vi "Check for change in Image Sizes.vi"(9 "Other optical path [Current ImRef]":T1, 10 "Current Optical Path [New ImRef]":T1, 11 "Current Optical Path [Current ImRef]":T1) -> (2 "Other Optical Path [New ImRef] OUT":T1, 3 "Current Optical Path [New ImRef] OUT":T1)   [LabVIEW 2012]
uses:
  <vilib>/vision/Image Controls.llb/IMAQ Image.ctl
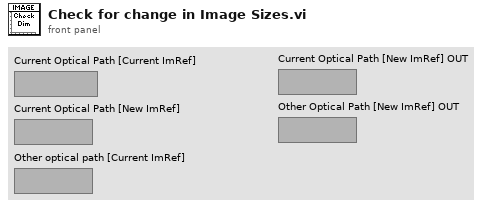
[diagram p1: front panel]
types:
  T1 = typedef "IMAQ Image.ctl" = refnum<image>
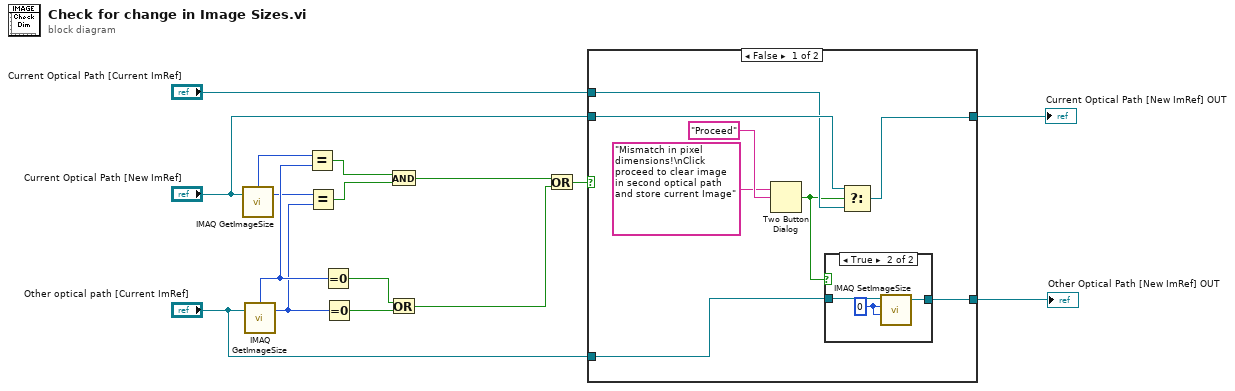
[diagram p0: block diagram]
diagram:
  n1 = call "IMAQ GetImageSize"("Image"="Current Optical Path [New ImRef]") -> ("Y Resolution"=w12:i32, "X Resolution"=w14:i32)  [unwired: 3 in, 1 out]
  n2 = call "IMAQ GetImageSize"("Image"="Other optical path [Current ImRef]") -> ("Y Resolution"=w11:i32, "X Resolution"=w13:i32)  [unwired: 3 in, 1 out]
  n3 = Equal?(x=w14, y=w13) -> (x = y?=w10:bool)
  n4 = Equal?(x=w12, y=w11) -> (x = y?=w9:bool)
  n5 = Equal To 0?(x=w13) -> (x = 0?=w16:bool)
  n6 = Equal To 0?(x=w11) -> (x = 0?=w15:bool)
  n7 = And(x=w10, y=w9) -> (x .and. y?=w8:bool)
  n8 = Or(x=w16, y=w15) -> (x .or. y?=w7:bool)
  n9 = Or(x=w8, y=w7) -> (x .or. y?=w6:bool)
  n10 = case shown="False" w6 {
    tunnel: "Current Optical Path [Current ImRef]" -> [w21 _]
    tunnel: "Current Optical Path [New ImRef]" -> [w22 w29]
    tunnel: "Other optical path [Current ImRef]" -> [w19 w30]
    tunnel: [w18 w30] -> w2
    tunnel: [w17 w29] -> w1
    frame False {
      n11 = Two Button Dialog(message="Mismatch in pixel dimensions!\nClick proceed to clear image in second optical path and store current Image", 2:"Proceed" ("T button name (\"OK\")")) -> (T button?=w20:bool)  [unwired: 1 in]
      n12 = case shown="True" w20 {
        tunnel: w19 -> [w25 w28]
        tunnel: [w25 w26] -> w18
        frame False {
        }
        frame True {
          w27 = 0 ("X Resolution")
          n13 = call "IMAQ SetImageSize"("Y Resolution"=w27, "X Resolution"=w27, "Image"=w28) -> ("Image Out"=w26:T1)  [unwired: 2 in, 1 out]
        }
      }
      n14 = Select(t=w22, s=w20, f=w21) -> (s? t:f=w17:T1)
    }
    frame True {
    }
  }
  "Current Optical Path [New ImRef] OUT" <- w1
  "Other Optical Path [New ImRef] OUT" <- w2
